vi "fnLasViewDrawWithFilterRight.vi"(1 "dWinSize":dbl, 2 "dSigma":dbl, 3 "pData":dbl[][](array[numeric])) -> (0 "返回类型":i32)   [LabVIEW 2012]
uses:
  LabView4Las.dll
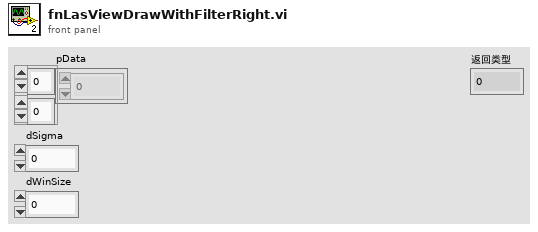
[diagram p1: front panel]
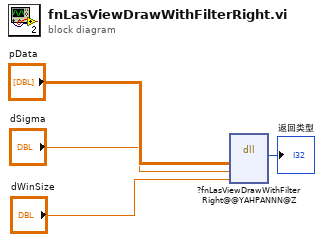
[diagram p0: block diagram]
diagram:
  n1 = dll-call lib="C:/Developer/labview/dll2/LabView4Las.dll" fn="?fnLasViewDrawWithFilterRight@@YAHPANNN@Z"("pData"="pData", "dSigma"="dSigma", "dWinSize"="dWinSize") -> ("返回类型"=→"返回类型":i32)  [unwired: 6 in, 2 out]
